vi "循环移位器.vi"() -> ()   [LabVIEW 2018]
panel:
  in  "确定按钮":bool
  out "Q3":bool
  out "Q2":bool
  out "Q1":bool
  out "Q0":bool
  in  "D3":bool
  in  "D2":bool
  in  "D0":bool
  in  "D1":bool
  in  "S1":bool
  in  "S0":bool
  in  "CLK":bool
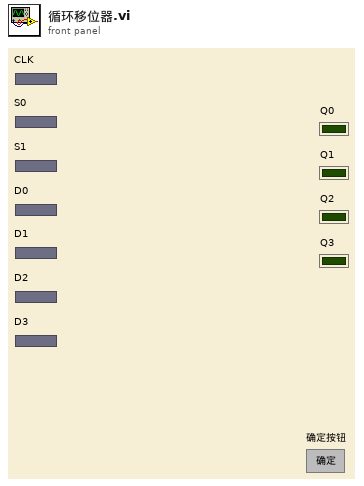
[diagram p1: front panel]
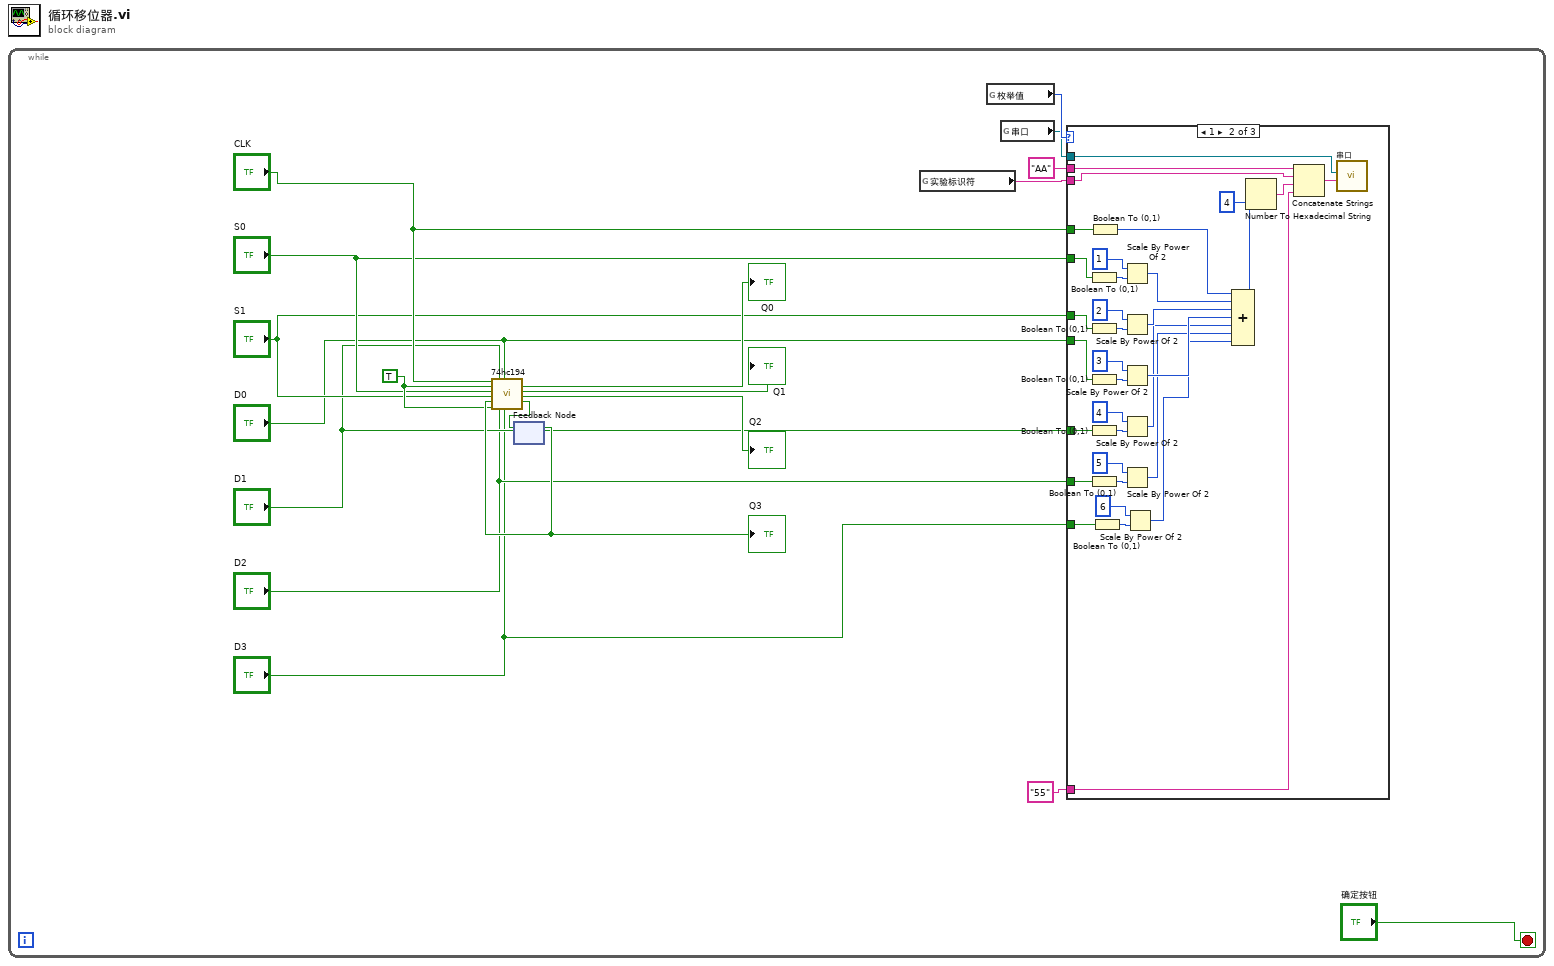
[diagram p0: block diagram]
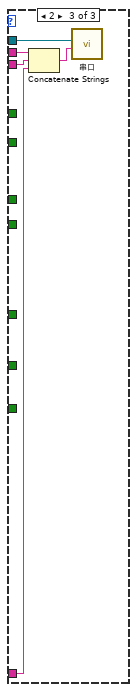
[diagram p3: hidden frame]
diagram:
  n1 = while {
    stop <- "确定按钮" stop-if-true
    w14 = TRUE
    n2 = feedback #1() -> (w15:bool)  [unwired: 1 in]
    "Q3" <- w15
    n3 = call "74hc194.vi"("cp"="CLK", "CR`"=w14, "S0"="S0", "S1"="S1", "Dsr"=w15, "Dsl"=w14, "D1"="D1", "D2"="D2", "D0"="D0", "D3"="D3") -> ("Q0"=→"Q0":bool, "Q1"=→"Q1":bool, "Q2"=→"Q2":bool, "Q3"=w16:bool)  [unwired: 6 in]
    n4 = feedback-in #1(w16) -> ()
    n5 = global read "全局变量.vi" "实验标识符"() -> (w10:string)
    n6 = global read "全局变量.vi" "枚举值"() -> (w12:i8)
    n7 = global read "全局变量.vi" "串口"() -> (w11:refnum<visa-resource-name>)
    n8 = case shown="1" w12 {
      tunnel: w11 -> [_ w48 w56]
      tunnel: w10 -> [_ w47 w57]
      tunnel: "55" -> [_ w46 w54]
      tunnel: "AA" -> [_ w45 w55]
      tunnel: "CLK" -> [_ w26 _]
      tunnel: "S0" -> [_ w25 _]
      tunnel: "S1" -> [_ w24 _]
      tunnel: "D0" -> [_ w23 _]
      tunnel: "D1" -> [_ w22 _]
      tunnel: "D2" -> [_ w21 _]
      tunnel: "D3" -> [_ w20 _]
      frame 0, Default {
      }
      frame 1 {
        n9 = Boolean To (0,1)(Boolean=w25) -> (0, 1=w50:i16)
        n10 = Boolean To (0,1)(Boolean=w24) -> (0, 1=w40:i16)
        n11 = Boolean To (0,1)(Boolean=w23) -> (0, 1=w38:i16)
        n12 = Boolean To (0,1)(Boolean=w22) -> (0, 1=w36:i16)
        n13 = Boolean To (0,1)(Boolean=w21) -> (0, 1=w34:i16)
        n14 = Boolean To (0,1)(Boolean=w26) -> (0, 1=w52:i16)
        n15 = Boolean To (0,1)(Boolean=w20) -> (0, 1=w29:i16)
        n16 = Scale By Power Of 2(n=1, x=w50) -> (x*2^n=w51:i16)
        n17 = Scale By Power Of 2(n=2, x=w40) -> (x*2^n=w41:i16)
        n18 = Scale By Power Of 2(n=3, x=w38) -> (x*2^n=w32:i16)
        n19 = Scale By Power Of 2(n=4, x=w36) -> (x*2^n=w31:i16)
        n20 = Scale By Power Of 2(n=5, x=w34) -> (x*2^n=w30:i16)
        n21 = Scale By Power Of 2(n=6, x=w29) -> (x*2^n=w27:i16)
        n22 = Compound Arithmetic op=ADD ("复合运算")(w52, w51, w41, w32, w31, w30, w27) -> (w44:i16)
        n23 = Number To Hexadecimal String(1:4, 2:w44) -> (0:w42:string)
        n24 = Concatenate Strings(w45, w47, w42, w46) -> (w53:string)
        n25 = call "串口.vi"("字符串"=w53, "VISA resource name"=w48) -> ()  [unwired: 10 in]
      }
      frame 2 {
        n26 = Concatenate Strings(w55, w57, w54) -> (w58:string)
        n27 = call "串口.vi"("字符串"=w58, "VISA resource name"=w56) -> ()  [unwired: 10 in]
      }
    }
  }
